vi "MatchFinder.vi"(10 "Start index":dbl, 11 "Frames":dbl[][](array[numeric])) -> (1 "Best Match":dbl, 3 "Utterance":dbl[](graph))   [LabVIEW 2013]
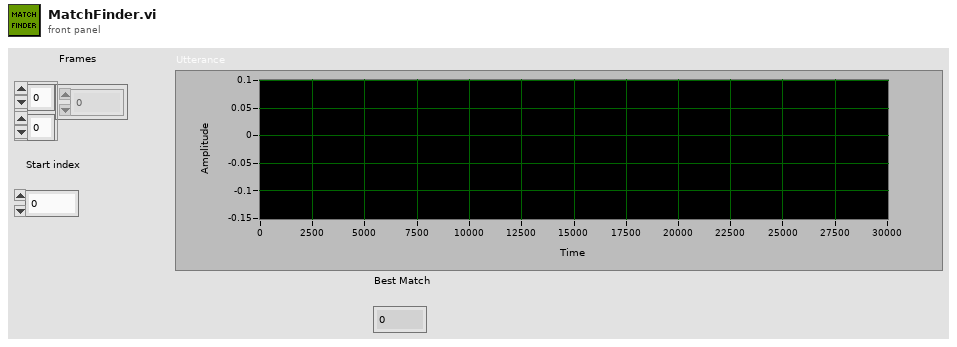
[diagram p1: front panel]
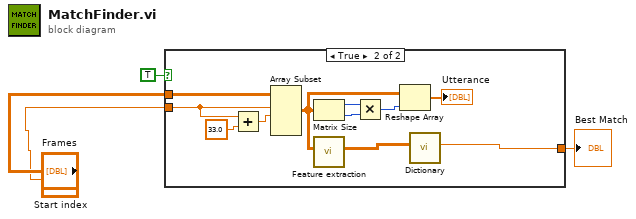
[diagram p0: block diagram]
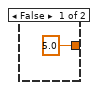
[diagram p2: hidden frame]
diagram:
  n1 = case shown="True" TRUE {
    tunnel: "Start index" -> [_ w9]
    tunnel: "Frames" -> [_ w10]
    tunnel: [5.0 ("Best Match") w8] -> w2
    frame False {
    }
    frame True {
      n2 = Add(x=w9, y=33.0 ("x")) -> (x+y=w15:dbl)
      n3 = Array Subset(array=w10, index (row)=w9, length (row)=w15) -> (w7:dbl[][])  [unwired: 2 in]
      n4 = Matrix Size(0:w7) -> (1:w14:i32, 2:w13:i32)
      n5 = call "Feature extraction.vi"("Utterance Frames"=w7) -> ("Acoustic vector"=w6:dbl[][])  [unwired: 10 in]
      n6 = Multiply(x=w14, y=w13) -> (x*y=w12:i32)
      n7 = Reshape Array(w7, w12) -> (→"Utterance":dbl[])
      n8 = call "Dictionary.vi"("Match Input"=w6) -> ("Best Match"=w8:dbl)  [unwired: 10 in]
    }
  }
  "Best Match" <- w2
